vi "畫ROI.vi"(8 "error in (no error)":errorcluster, 10 "ROI In":T1, 11 "Image In":T2) -> (0 "error out":errorcluster, 2 "ROI out":T1, 3 "Image":T2(plugin-control))   [LabVIEW 2015]
uses:
  <vilib>/vision/Image Controls.llb/IMAQ Image.ctl
panel:
  in  "Path":path
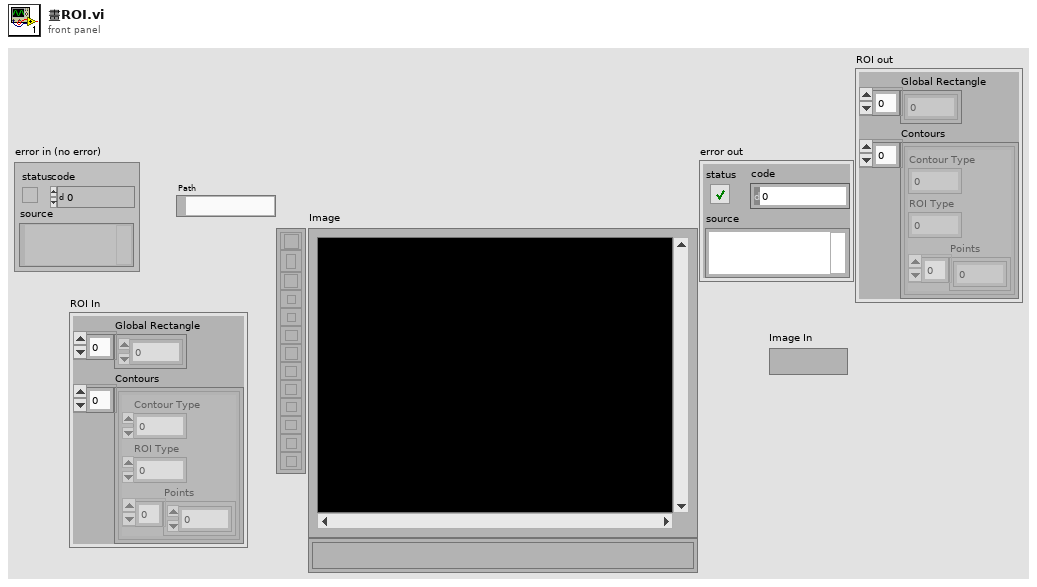
[diagram p1: front panel]
types:
  T1 = cluster{"Global Rectangle":i32[], "Contours":cluster{"Contour Type":u32, "ROI Type":u32, "Points":i32[]}[]}
  T2 = typedef "IMAQ Image.ctl" = refnum<image>
  T3 = cluster{"Contour Type":u32, "ROI Type":u32, "Points":i32[]}[]
  T4 = cluster{"Contour Type":u32, "ROI Type":u32, "Points":i32[]}
  T5 = typedef "ROI Descriptor" = cluster{"Global Rectangle":i32[], "Contours":cluster{"ID":enum32{"External", "Internal"}, "Type":u32, "Coordinates":i32[]}[]}
  T6 = cluster{"Left":i32, "Top":i32, "Right":i32, "Bottom":i32}
  T7 = typedef "IMAQ Line" = cluster{"Start X":i32, "Start Y":i32, "End X":i32, "End Y":i32}
  T8 = typedef "IMAQ Rectangle" = cluster{"Left":i32, "Top":i32, "Right":i32, "Bottom":i32, "Rotation":dbl}
  T9 = cluster{"Points[0]":i32, "Points[1]":i32, "Points[2]":i32, "Points[3]":i32, "Points[4]":i32}
  T10 = typedef "IMAQ Circle" = cluster{"Center X":i32, "Center Y":i32, "Inner Radius":i32, "Outer Radius":i32, "Start Angle":dbl, "End Angle":dbl}
  T11 = typedef "IMAQ Point" = cluster{"X":sgl, "Y":sgl}
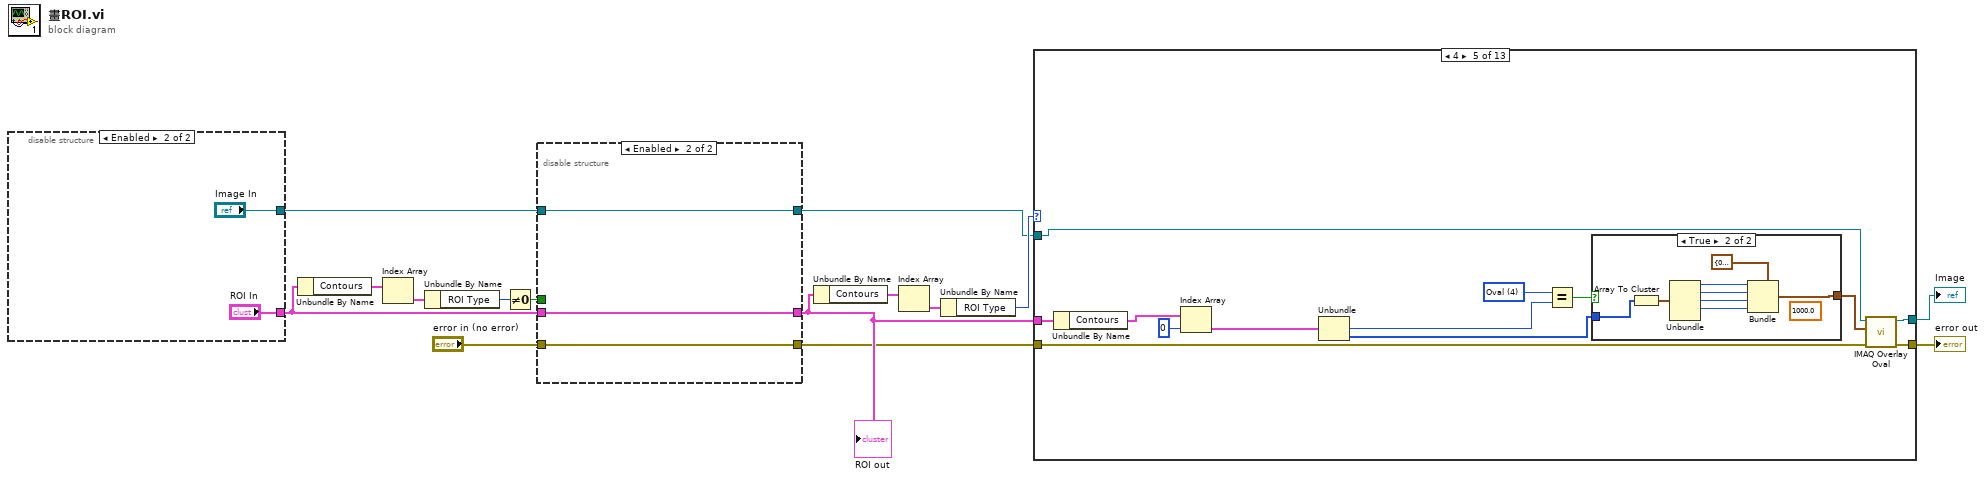
[diagram p0: block diagram]
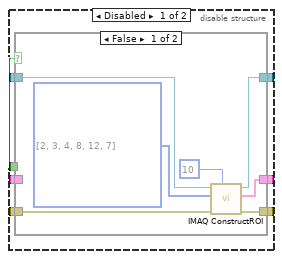
[diagram p2: hidden frame]
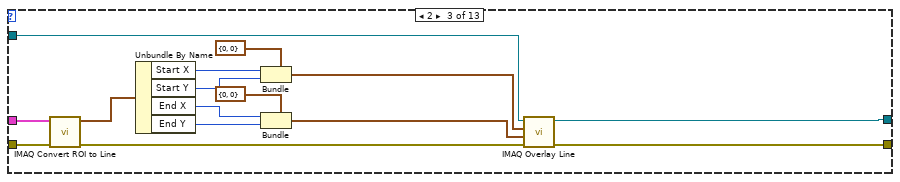
[diagram p6: hidden frame]
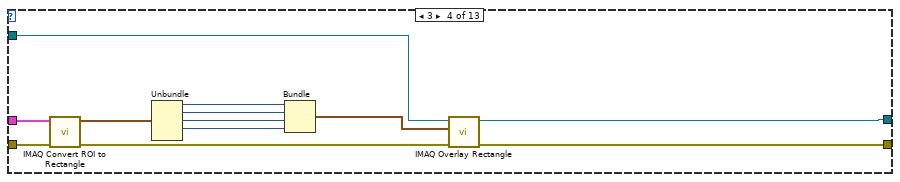
[diagram p7: hidden frame]
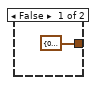
[diagram p8: hidden frame]
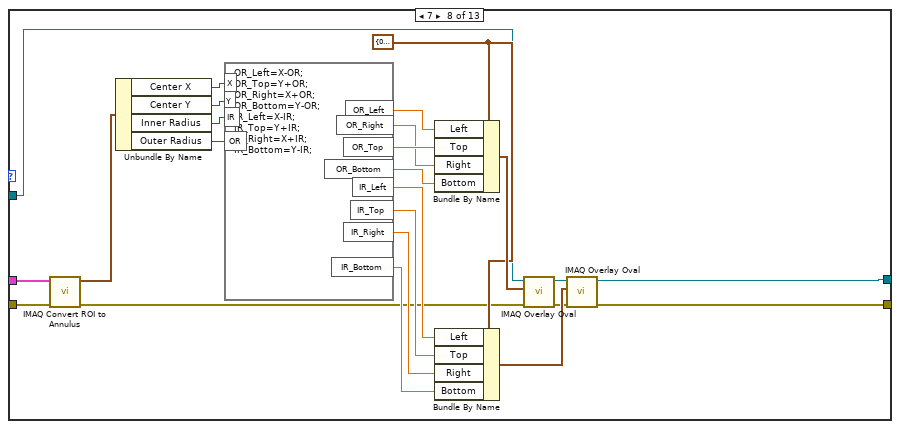
[diagram p11: hidden frame]
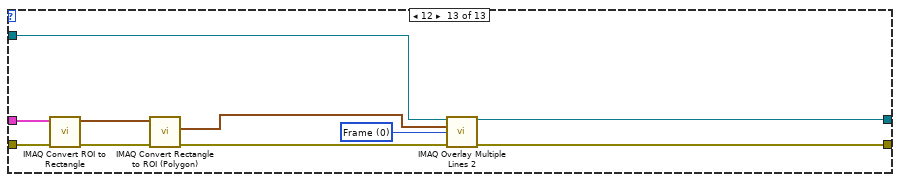
[diagram p16: hidden frame]
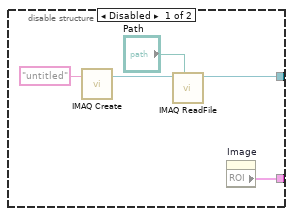
[diagram p17: hidden frame]
diagram:
  n1 = disable-structure shown="Enabled" {
    disable-tunnel: [w17 "Image In"] -> w6
    disable-tunnel: [w16 "ROI In"] -> w1
    frame Disabled {
      n2 = call "IMAQ Create"("Image Name"="untitled") -> ("New Image"=w19:T2)  [unwired: 4 in, 1 out]
      n3 = call "IMAQ ReadFile"("File Path"="Path", "Image"=w19) -> ("Image Out"=w17:T2)  [unwired: 5 in, 4 out]
      n4 = property on="Image" class="ImageControl"() -> ("ROI"=w16:T1)  [unwired: 2 in, 2 out]
    }
    frame Enabled {
    }
  }
  n5 = Unbundle By Name(w1) -> ("Contours"=w10:T3)
  n6 = Index Array(array=w10) -> (element=w9:T4)  [unwired: 1 in]
  n7 = Unbundle By Name(w9) -> ("ROI Type"=w8:u32)
  n8 = Not Equal To 0?(x=w8) -> (x != 0?=w7:bool)
  n9 = disable-structure shown="Enabled" {
    disable-tunnel: w7 -> [w29 _]
    disable-tunnel: w6 -> [w28 w42]
    disable-tunnel: [w27 w42] -> w5
    disable-tunnel: [w26 w41] -> w4
    disable-tunnel: "error in (no error)" -> [w25 w40]
    disable-tunnel: [w24 w40] -> w2
    disable-tunnel: w1 -> [w23 w41]
    frame Disabled {
      n10 = case shown="False" w29 {
        tunnel: [w34 w39] -> w26
        tunnel: w23 -> [_ w39]
        tunnel: w28 -> [w33 w38]
        tunnel: [w32 w38] -> w27
        tunnel: w25 -> [w31 w37]
        tunnel: [w30 w37] -> w24
        frame False {
          w36 = u32[] [2, 3, 4, 8, 12, 7] items=["No Selection", "Point", "Line", "Rectangle", "Oval", "Polygon", "Freehand Region", "Annulus", "Zoom", "Pan", "Broken Line", "Freehand Line", "Rotated Rectangle"] ("Tools")
          n11 = call "IMAQ ConstructROI"("Window Number (-1...15)"=10, "error in (no error)"=w31, "Tools"=w36, "Image"=w33) -> ("error out"=w30:errorcluster, "ROI Descriptor Out"=w34:T5, "Image Out (duplicate)"=w32:T2)  [unwired: 4 in, 1 out]
        }
        frame True {
        }
      }
    }
    frame Enabled {
    }
  }
  "ROI out" <- w4
  n12 = Unbundle By Name(w4) -> ("Contours"=w15:T3)
  n13 = Index Array(array=w15) -> (element=w14:T4)  [unwired: 1 in]
  n14 = Unbundle By Name(w14) -> ("ROI Type"=w12:u32)
  n15 = case shown="4" w12 {
    tunnel: w5 -> [w44 _ w59 w71 w84 _ _ w99 _ _ _ _ w123]
    tunnel: [w44 _ w58 w70 w83 _ _ w105 _ _ _ _ w122] -> w13
    tunnel: w4 -> [_ _ w53 w63 w81 _ _ w107 _ _ _ _ w127]
    tunnel: w2 -> [w43 _ w45 w62 w73 _ _ w97 _ _ _ _ w121]
    tunnel: [w43 _ w47 w60 w72 _ _ w94 _ _ _ _ w118] -> w11
    frame 0, Default {
    }
    frame 1 {
    }
    frame 2 {
      n16 = call "IMAQ Convert ROI to Line"("error in (no error)"=w45, "ROI Descriptor"=w53) -> ("error out"=w46:errorcluster, "Line"=w52:T7)  [unwired: 7 in]
      n17 = Unbundle By Name(w52) -> ("Start X"=w50:i32, "Start Y"=w51:i32, "End X"=w49:i32, "End Y"=w48:i32)
      n18 = Bundle(cluster=cluster{"X":i32, "Y":i32} {"X"=0, "Y"=0} ("Start Point"), "X"=w50, "Y"=w51) -> (w56:cluster{"X":i32, "Y":i32})
      n19 = Bundle(cluster=cluster{"X":i32, "Y":i32} {"X"=0, "Y"=0} ("Start Point"), "X"=w49, "Y"=w48) -> (w57:cluster{"X":i32, "Y":i32})
      n20 = call "IMAQ Overlay Line"("error in (no error)"=w46, "End Point"=w57, "Start Point"=w56, "Image"=w59) -> ("error out"=w47:errorcluster, "Image Out"=w58:T2)  [unwired: 6 in]
    }
    frame 3 {
      n21 = call "IMAQ Convert ROI to Rectangle"("error in (no error)"=w62, "ROI Descriptor"=w63) -> ("error out"=w61:errorcluster, "Rectangle"=w65:T8)  [unwired: 7 in]
      n22 = Unbundle(w65) -> ("Left"=w66:i32, "Top"=w67:i32, "Right"=w68:i32, "Bottom"=w69:i32)  [unwired: 1 out]
      n23 = Bundle("Left"=w66, "Top"=w67, "Right"=w68, "Bottom"=w69) -> (w64:T6)  [unwired: 1 in]
      n24 = call "IMAQ Overlay Rectangle"("error in (no error)"=w61, "Rectangle"=w64, "Image"=w71) -> ("error out"=w60:errorcluster, "Image Out"=w70:T2)  [unwired: 7 in]
    }
    frame 4 {
      w75 = u32 4 items=["No Selection", "Point", "Line", "Rectangle", "Oval", "Polygon", "Free", "Annulus", "Unused2", "Unused3", "Broken Line", "Free Hand Line", "Rotated Rectangle"] ("Type")
      n25 = Unbundle By Name(w81) -> ("Contours"=w77:T3)
      n26 = Index Array(array=w77, index=0 ("Index")) -> (element=w79:T4)
      n27 = Unbundle(w79) -> ("ROI Type"=w76:u32, "Points"=w78:i32[])  [unwired: 1 out]
      n28 = Equal?(x=w75, y=w76) -> (x = y?=w74:bool)
      n29 = case shown="True" w74 {
        tunnel: w78 -> [_ w93]
        tunnel: [T6 {"Left"=0, "Top"=0, "Right"=0, "Bottom"=0} ("Bounding Rectangle") w86] -> w82
        frame False {
        }
        frame True {
          (unwired) 1000.0 ("y")
          n30 = Array To Cluster(array=w93) -> (cluster=w92:T9)
          n31 = Unbundle(w92) -> ("Points[0]"=w91:i32, "Points[1]"=w90:i32, "Points[2]"=w89:i32, "Points[3]"=w88:i32)  [unwired: 1 out]
          n32 = Bundle(cluster=T6 {"Left"=0, "Top"=0, "Right"=0, "Bottom"=0} ("Bounding Rectangle"), "Left"=w91, "Top"=w90, "Right"=w89, "Bottom"=w88) -> (w86:T6)
        }
      }
      n33 = call "IMAQ Overlay Oval"("error in (no error)"=w73, "Bounding Rectangle"=w82, "Image"=w84) -> ("error out"=w72:errorcluster, "Image Out"=w83:T2)  [unwired: 7 in]
    }
    frame 5 {
    }
    frame 6 {
    }
    frame 7 {
      w104 = T6 {"Left"=0, "Top"=0, "Right"=0, "Bottom"=0} ("Bounding Rectangle")
      n34 = call "IMAQ Convert ROI to Annulus"("error in (no error)"=w97, "ROI Descriptor"=w107) -> ("error out"=w96:errorcluster, "Annulus"=w117:T10)  [unwired: 7 in]
      n35 = Unbundle By Name(w117) -> ("Center X"=w116:i32, "Center Y"=w115:i32, "Inner Radius"=w114:i32, "Outer Radius"=w113:i32)
      n36 = formula code="OR_Left=X-OR;\nOR_Top=Y+OR;\nOR_Right=X+OR;\nOR_Bottom=Y-OR;\nIR_Left=X-IR;\nIR_Top=Y+IR;\nIR_Right=X+IR;\nIR_Bottom=Y-IR;"("X"=w116, "Y"=w115, "IR"=w114, "OR"=w113) -> ("OR_Left"=w110:dbl, "OR_Right"=w111:dbl, "OR_Top"=w112:dbl, "OR_Bottom"=w109:dbl, "IR_Left"=w103:dbl, "IR_Top"=w102:dbl, "IR_Right"=w101:dbl, "IR_Bottom"=w100:dbl)
      n37 = Bundle By Name(cluster=w104, "Left"=w110, "Top"=w112, "Right"=w111, "Bottom"=w109) -> (w108:T6)
      n38 = Bundle By Name(cluster=w104, "Left"=w103, "Top"=w102, "Right"=w101, "Bottom"=w100) -> (w106:T6)
      n39 = call "IMAQ Overlay Oval"("error in (no error)"=w96, "Bounding Rectangle"=w108, "Image"=w99) -> ("error out"=w95:errorcluster, "Image Out"=w98:T2)  [unwired: 7 in]
      n40 = call "IMAQ Overlay Oval"("error in (no error)"=w95, "Bounding Rectangle"=w106, "Image"=w98) -> ("error out"=w94:errorcluster, "Image Out"=w105:T2)  [unwired: 7 in]
    }
    frame 8 {
    }
    frame 9 {
    }
    frame 10 {
    }
    frame 11 {
    }
    frame 12 {
      w124 = u32 0 items=["Frame", "Fill"] ("Drawing Mode (Frame)")
      n41 = call "IMAQ Convert ROI to Rectangle"("error in (no error)"=w121, "ROI Descriptor"=w127) -> ("error out"=w120:errorcluster, "Rectangle"=w126:T8)  [unwired: 7 in]
      n42 = call "IMAQ Convert Rectangle to ROI (Polygon)"("error in (no error)"=w120, "Rectangle"=w126) -> ("error out"=w119:errorcluster, "Rectangle Points"=w125:T11[])  [unwired: 6 in, 1 out]
      n43 = call "IMAQ Overlay Multiple Lines 2"("Image"=w123, "Line End Points"=w125, "Drawing Mode (Frame)"=w124, "error in (no error)"=w119) -> ("Image Out"=w122:T2, "error out"=w118:errorcluster)  [unwired: 10 in]
    }
  }
  "Image" <- w13
  "error out" <- w11
